vi "Get Trigger Information.vi"(10 "level":dbl format="%.2p", 11 "Waveform":waveform(dbl)) -> (3 "Trigger Information":T1)   [LabVIEW 2015, in "Exposure Process.lvlib"]
uses:
  Exposure Process.lvlib
  Control_Start-End-Trigger.ctl
  <vilib>/measure/mamon.llb/Trigger Detection for 1 Channel.vi
  <vilib>/Waveform/WDTOps.llb/WDT Get Waveform Subset DBL.vi
  <vilib>/measure/NI_MAPro.lvlib
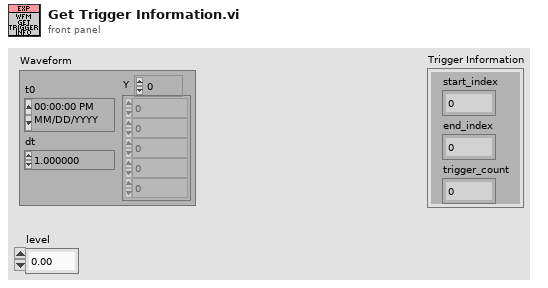
[diagram p1: front panel]
types:
  T1 = typedef "Exposure Process.lvlib/Control_Start-End-Trigger.ctl" = cluster{"start_index":i64, "end_index":i64, "trigger_count":i64}
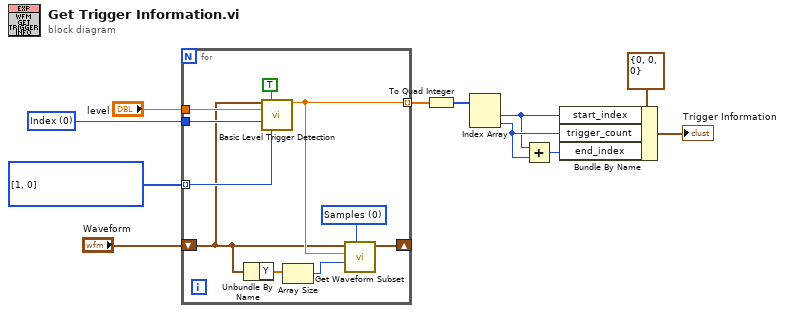
[diagram p0: block diagram]
diagram:
  w8 = u16 0 items=["Index", "Time"] ("location mode")
  w10 = u16[] [1, 0] items=["Falling Edge", "Rising Edge"]
  n1 = for {
    tunnel: w10 -> [w20] mode=indexing
    tunnel: "level" -> [w19]
    shift-right: [w17] -> _
    shift-left: "Waveform" -> [w14]
    tunnel: w8 -> [w18]
    tunnel: [w15] -> w6 mode=indexing
    w16 = u16 0 items=["Samples", "Relative Time"] ("start/duration format")
    n2 = Unbundle By Name(w14) -> ("Y"=w13:dbl[])
    n3 = call-poly <vilib>:"Basic Level Trigger Detection.vi"("signal in"=w14, "reset"=TRUE, "level"=w19, "location mode"=w18, "trigger slope"=w20) -> ("trigger location"=w15:dbl)  [unwired: 8 in, 2 out]
    n4 = Array Size(array=w13) -> (size(s)=w12:i32)
    n5 = call-poly <vilib>:"Get Waveform Subset.vi"("start/duration format"=w16, "duration"=w12, "start samples/time"=w15, "waveform in"=w14) -> ("waveform out"=w17:waveform(dbl))  [unwired: 2 in, 3 out]
  }
  n6 = To Quad Integer(1:w6) -> (0:w5:i64[])
  n7 = Index Array(array=w5) -> (element #1=w2:i64, element #2=w3:i64)  [unwired: 2 in]
  n8 = Add(x=w2, y=w3) -> (x+y=w4:i64)
  n9 = Bundle By Name(cluster=T1 {"start_index"=0, "end_index"=0, "trigger_count"=0} ("Cluster"), "start_index"=w2, "trigger_count"=w3, "end_index"=w4) -> (→"Trigger Information":T1)
